vi "SwerveJoystickStrafeScaling.vi"(0 "Raw Joystick X":dbl, 5 "Raw Joystick Y":dbl, 7 "Auto Control":bool, 9 "Strafe Deadband":dbl(slide)=0.05 min=0.0 max=0.25 scale=0.0..0.25, 11 "Strafe Scaling":dbl(slide)=2.0 min=1.0 max=4.0 scale=1.0..4.0, 12 "Strafe Maximum":dbl(slide)=1.0 min=0.3 max=1.0 scale=0.3..1.0) -> (4 "In Deadband":bool, 8 "Scaled Joystick X":dbl format="%.2f", 15 "Scaled Joystick Y":dbl format="%.2f")   [LabVIEW 2020]
doc: "Applies a deadband and nonlinear scaling to the strafe axes of a swerve drive. Includes a hook to override the non-linear deadband and scaling when the rotation is under autonomous control. Includes a de-saturation check to handle compounding drive commands from different controllers (e.g. direct driver control + auto targeting)."
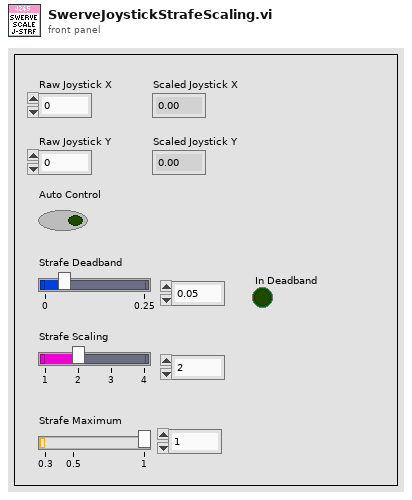
[diagram p1: front panel]
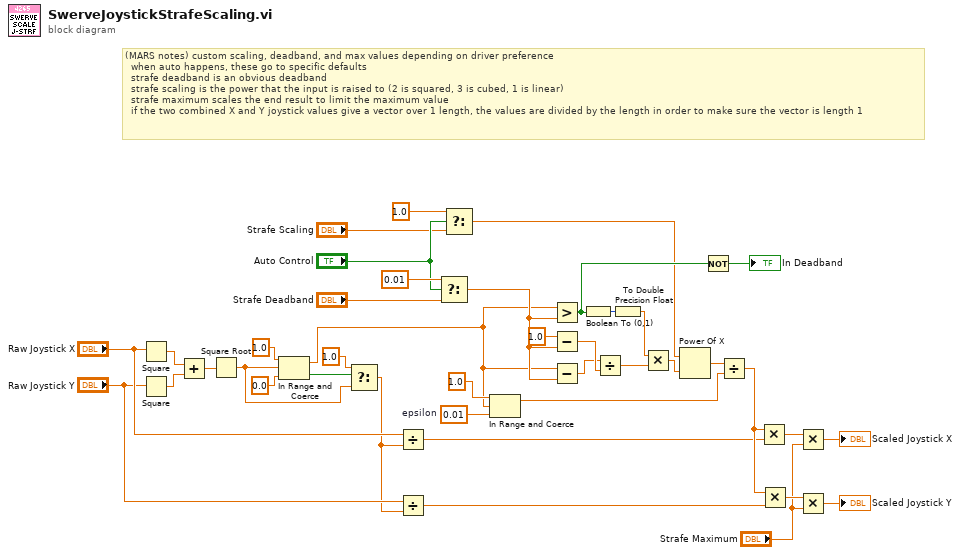
[diagram p0: block diagram]
diagram:
  w35 = 0.01  # epsilon
  # "(MARS notes) custom scaling, deadband, and max values depending on driver preference\n\t\twhen auto happens, these go to specific defaults\n\t\tstrafe deadband is an obvious deadband\n\t\tstrafe scaling is the power that the input is raised to (2 is squared, 3 is cubed, 1 is linear)\n\t\tstrafe maximum scales the end result to limit the maximum value\n\t\tif the two combined X and Y joystick values give a vector over 1 length, the values are divided by the length in order to make sure the vector is length 1"
  n1 = Square(x="Raw Joystick X") -> (x^2=w32:dbl)
  n2 = Square(x="Raw Joystick Y") -> (x^2=w31:dbl)
  n3 = Add(x=w32, y=w31) -> (x+y=w33:dbl)
  n4 = Square Root(x=w33) -> (sqrt(x)=w12:dbl)
  n5 = In Range and Coerce(upper limit=1.0, x=w12, lower limit=0.0 ("upper limit")) -> (coerced(x)=w6:dbl, In Range?=w14:bool)
  n6 = Select(t=1.0, s=w14, f=w12) -> (s? t:f=w7:dbl)
  n7 = Divide(x="Raw Joystick X", y=w7) -> (x/y=w11:dbl)
  n8 = Divide(x="Raw Joystick Y", y=w7) -> (x/y=w8:dbl)
  n9 = Select(t=0.01, s="Auto Control", f="Strafe Deadband") -> (s? t:f=w17:dbl)
  n10 = Select(t=1.0, s="Auto Control", f="Strafe Scaling") -> (s? t:f=w18:dbl)
  n11 = In Range and Coerce(upper limit=1.0, x=w6, lower limit=w35) -> (coerced(x)=w34:dbl)  [unwired: 1 out]
  n12 = Greater?(x=w6, y=w17) -> (0:w38:bool)
  n13 = Subtract(x=1.0, y=w17) -> (x-y=w29:dbl)
  n14 = Subtract(x=w6, y=w17) -> (x-y=w27:dbl)
  n15 = Boolean To (0,1)(Boolean=w38) -> (0, 1=w25:i16)
  n16 = Divide(x=w27, y=w29) -> (x/y=w30:dbl)
  n17 = To Double Precision Float(number=w25) -> (double precision float=w26:dbl)
  n18 = Multiply(x=w26, y=w30) -> (x*y=w39:dbl)
  n19 = Power Of X(1:w39, 2:w18) -> (0:w40:dbl)
  n20 = Not(x=w38) -> (.not. x?=→"In Deadband":bool)
  n21 = Divide(x=w40, y=w34) -> (x/y=w37:dbl)
  n22 = Multiply(x=w37, y=w11) -> (x*y=w4:dbl)
  n23 = Multiply(x=w37, y=w8) -> (x*y=w5:dbl)
  n24 = Multiply(x=w4, y="Strafe Maximum") -> (x*y=→"Scaled Joystick X":dbl)
  n25 = Multiply(x=w5, y="Strafe Maximum") -> (x*y=→"Scaled Joystick Y":dbl)
